vi "resmeas.vi"(9 "Rc":dbl caption="Contact resistance", 10 "Im":dbl=0.00395, 11 "Um":dbl=0.00395) -> (3 "Rm":dbl)   [LabVIEW 2014]
doc: "DAQ kártya segítségével szondaellenállást mér egy kalibrált feszültség (Calibrated Voltage) segítségével beállított mérõ áram (Im) mellett, megadott TK segítségével átszámítja a mért ellenállás értéket Tnom-on mértre (Rm,nom), majd a megadott elvárt ellenállás (Required Resistance) és annak toleranciája (Resistance Tolerance) alapján javaslatot tesz, hogy milyen tartományba esõ sönt ellenállással (Rcorr,min...Rcorr,max) lehet az ellenállásértéket a kívánt tartományba húzni. Ha nem lehet, vagy nem kell, vagy gyanúsan magas ellenállást mér, akkor megfelelõ jelzést ad (Fail, Final OK, High R). Ha nem sikerült beállítani a kívánt mérõáramot, akkor jelzi ezt (Adj Failed) és nem hajtja végre a mérést. A mért hõmérsékletet az Acquired Temperature kimeneten kapjuk meg °C-ban. Resister values = [Rm; Rm,nom; Rcorr,min; Rcorr,max]"
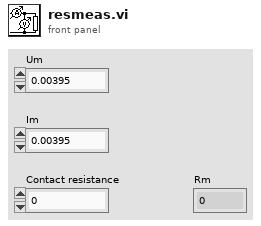
[diagram p1: front panel]
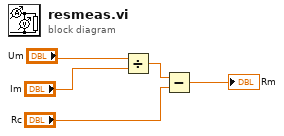
[diagram p0: block diagram]
diagram:
  n1 = Divide(x="Um", y="Im") -> (x/y=w5:dbl)
  n2 = Subtract(x=w5, y="Rc") -> (x-y=→"Rm":dbl)
